vi "CallTestSuiteMethod.vi"(8 "error in":errorcluster, 10 "method":T1, 11 "TestSuite in":refnum<class "TestSuite.lvclass">) -> (0 "error out":errorcluster, 2 "Test Method Error":errorcluster, 3 "TestSuite out":refnum<class "TestSuite.lvclass">)   [LabVIEW 2011, in "TestSuite.lvclass"]
uses:
  TestSuite.lvclass
  Method--enum.ctl
  TestSuite.lvclass/TestSuite.ctl
  JKI Reuse/Filter Error Codes (Scalar)__jki_lib_error_handling -- VI Tester.vi
  Libraries/VITesterUtilities.lvlib
panel:
  # "JKI VI Tester for LabVIEW\nhttp://jkisoft.com/vi-tester\nCopyright (C) 2007-2009, JKI <info@jkisoft.com>\nALL RIGHTS RESERVED"
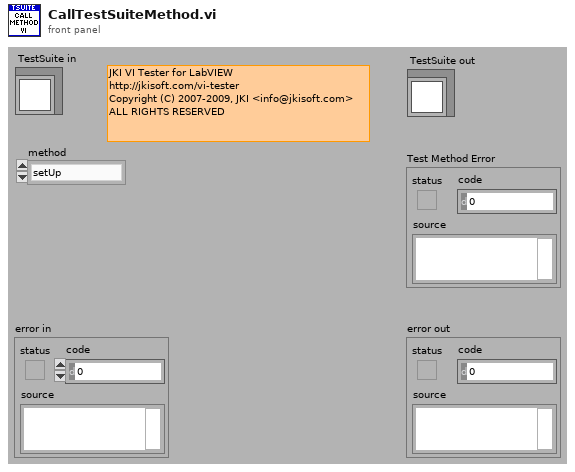
[diagram p1: front panel]
types:
  T1 = typedef "TestSuite.lvclass/Method--enum.ctl" = enum16{"setUp", "tearDown"}
  T2 = enum32{"Bad", "Idle", "Run top level", "Running"}
  T3 = cluster{"name":string, "type desc":i16[], "flat data":string}
  T4 = cluster{"name":string, "type desc":i16[], "flat data":string}[]
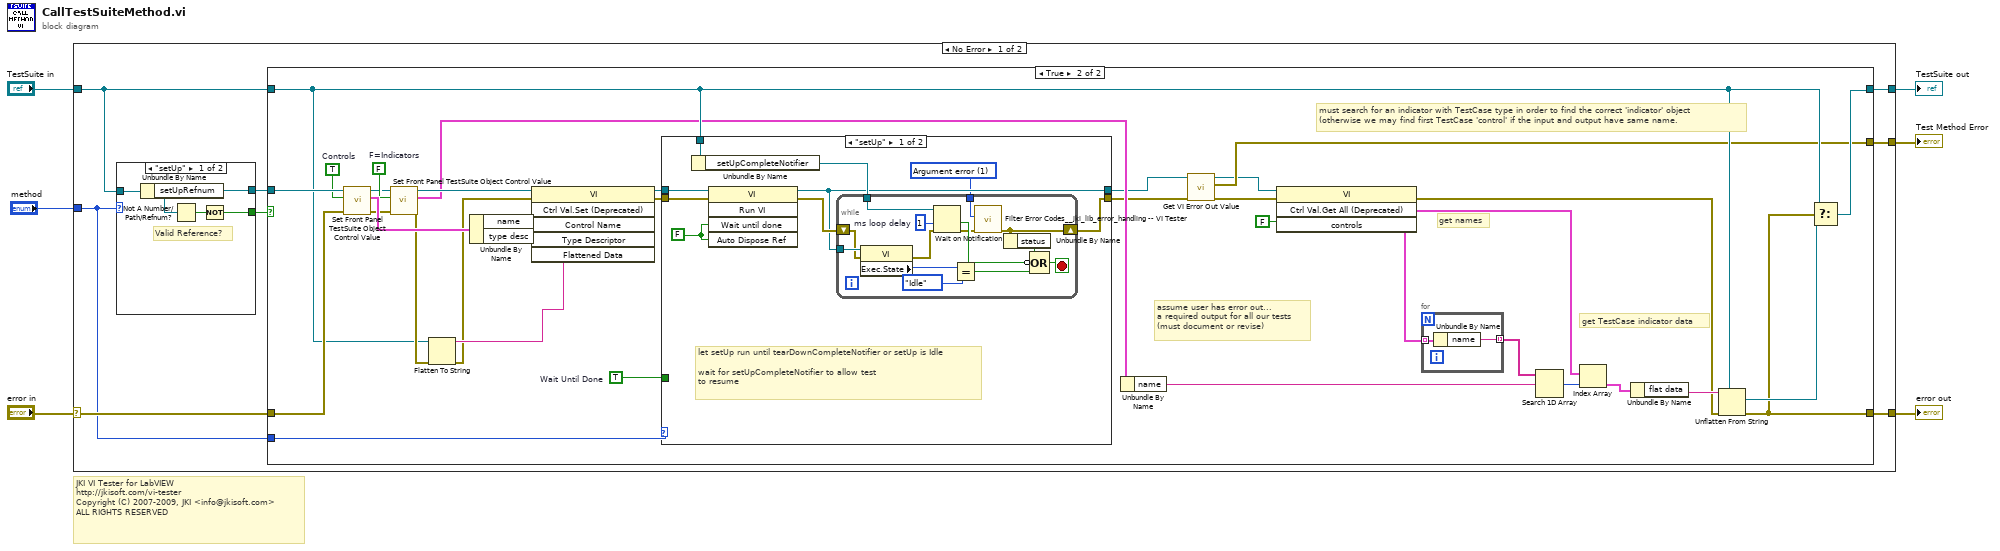
[diagram p0: block diagram]
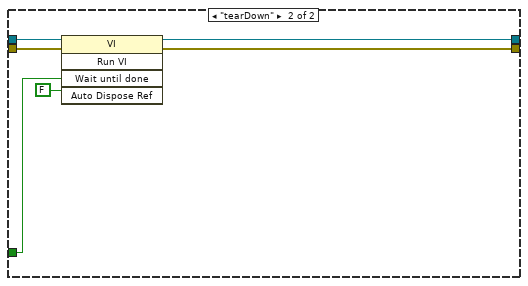
[diagram p3: hidden frame]
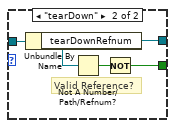
[diagram p4: hidden frame]
diagram:
  # "JKI VI Tester for LabVIEW\nhttp://jkisoft.com/vi-tester\nCopyright (C) 2007-2009, JKI <info@jkisoft.com>\nALL RIGHTS RESERVED"
  n1 = case shown="No Error" "error in" {
    selector: "error in" -> [w9 w92]
    tunnel: [w14 w91] -> w2
    tunnel: [w13 _] -> w3
    tunnel: [w12 w92] -> w4
    tunnel: "TestSuite in" -> [w11 w91]
    tunnel: "method" -> [w7 _]
    frame No Error {
      n2 = case shown="\"setUp\"" w7 {
        tunnel: w11 -> [w86 w90]
        tunnel: [w85 w89] -> w10
        tunnel: [w83 w87] -> w8
        frame "setUp" {
          # "Valid Reference?"
          n3 = Unbundle By Name(w86) -> ("setUpRefnum"=w85:refnum<vi>)
          n4 = Not A Number/Path/Refnum?(number/path/refnum=w85) -> (NaN/Path/Refnum?=w84:bool)
          n5 = Not(x=w84) -> (.not. x?=w83:bool)
        }
        frame "tearDown" {
          # "Valid Reference?"
          n6 = Unbundle By Name(w90) -> ("tearDownRefnum"=w89:refnum<vi>)
          n7 = Not A Number/Path/Refnum?(number/path/refnum=w89) -> (NaN/Path/Refnum?=w88:bool)
          n8 = Not(x=w88) -> (.not. x?=w87:bool)
        }
      }
      n9 = case shown="True" w8 {
        tunnel: [w16 w51] -> w14
        tunnel: [_ w18] -> w13
        tunnel: [w15 w26] -> w12
        tunnel: w11 -> [w16 w29]
        tunnel: w10 -> [_ w47]
        tunnel: w9 -> [w15 w38]
        tunnel: w7 -> [_ w35]
        frame False {
        }
        frame True {
          w34 = TRUE  # Wait Until Done
          w42 = FALSE  # F=Indicators
          w46 = TRUE  # Controls
          # "get TestCase indicator data"
          # "get names"
          # "must search for an indicator with TestCase type in order to find the correct 'indicator' object\n(otherwise we may find first TestCase 'control' if the input and output have same name."
          # "assume user has error out...\na required output for all our tests\n(must document or revise)"
          n10 = call "Set Front Panel TestSuite Object Control Value.vi"("error in"=w38, "Control (F: Indicator)"=w46, "vi reference"=w47) -> ("error out"=w41:errorcluster, "Control Value"=w45:T3, "dup vi reference"=w40:refnum<vi>)  [unwired: 5 in, 1 out]
          n11 = call "Set Front Panel TestSuite Object Control Value.vi"("error in"=w41, "Control (F: Indicator)"=w42, "vi reference"=w40) -> ("error out"=w37:errorcluster, "Control Value"=w25:T3, "dup vi reference"=w39:refnum<vi>)  [unwired: 5 in, 1 out]
          n12 = Flatten To String(anything=w29, error in (no error)=w37) -> (data string=w48:string, error out=w36:errorcluster)  [unwired: 2 in, 1 out]
          n13 = Unbundle By Name(w45) -> ("name"=w44:string, "type desc"=w43:i16[])
          n14 = invoke class="VI" method="Ctrl Val.Set (Deprecated)"(reference=w39, error in=w36, "Control Name"=w44, "Type Descriptor"=w43, "Flattened Data"=w48) -> (reference out=w50:refnum<vi>, error out=w49:errorcluster)  [unwired: 1 in, 4 out]
          n15 = case shown="\"setUp\"" w35 {
            tunnel: w50 -> [w62 w82]
            tunnel: w49 -> [w61 w81]
            tunnel: [w55 w80] -> w21
            tunnel: [w56 w79] -> w20
            tunnel: w34 -> [_ w77]
            tunnel: w29 -> [w59 _]
            frame "setUp" {
              w54 = 1 items=["No error", "Argument error", "Memory is full", "Out of zone", "End of file", "File already open", "Generic file I/O error", "File not found", "File permission error", "Disk is full", "Duplicate path", "Too many files open", "System feature not enabled", "Resource file not found", "Cannot add resource", "Resource not found", "Image not found", "Image memory error", "Pen does not exist", "Config type invalid", "Config token not found", "Config parse error", "Config memory error", "Bad external code format", "Bad external code offset", "External code not present", "Null window", "Destroy window error", "Null menu", "Print aborted", "Bad print record", "Print driver error", "Windows error during printing", "Memory error during printing", "Print dialog error", "Generic print error", "Invalid device refnum", "Device not found", "Device parameter error", "Device unit error", "Cannot open device", "Device call aborted", "Generic error", "Cancelled by user", "Object ID too low", "Object ID too high", "Object not in heap", "Unknown heap", "Unknown object (invalid DefProc)", "Unknown object (DefProc not in table)", "Message out of range", "Invalid (null) method", "Unknown message", "Manager call not supported", "Bad address", "Network operation in progress", "Network operation timed out", "Connection is busy", "Network attribute not supported", "Network error", "Address in use", "System out of memory", "Connection aborted", "Connection refused", "Not connected", "Already connected", "Connection closed", "Initialization error (interapplication manager)", "Bad occurrence", "Wait on unbound occurrence handler", "Occurrence queue overflow", "Datalog type conflict", "Unused", "Unrecognized type (interapplication manager)", "Memory corrupt", "Failed to make temporary DLL", "Old CIN version", "Drag socket not found", "Failed to load drop-object", "Failed to register OLE object", "Failed to release OLE object", "Format specifier type mismatch", "Unknown format specifier", "Too few format specifiers", "Too many format specifiers", "Scan failed", "Newer CIN version", "Error converting to variant", "Runtime menu error", "Password tampered", "Variant attribute not found", "Incompatible variant data type", "Event data is not available", "Event Store is not present", "Occurrence is not found", "Event Queue is not created", "Event info is not available", "Refnum passed is NULL", "Error retrieving Class GUID", "Error retrieving CoClass GUID", "Error retrieving TypeLib GUID.", "Bad built application magic bytes.", "Specific driver is different from the specific driver associated with the Logical Name.", "There is no session opened to the class driver.", "Max Error", "MAX - Error with config objects", "MAX - Error loading configuration", "MAX - Group not supported"]
              w60 = FALSE ("Auto Dispose Reference")
              # "let setUp run until tearDownCompleteNotifier or setUp is Idle\n\nwait for setUpCompleteNotifier to allow test\nto resume"
              n16 = Unbundle By Name(w59) -> ("setUpCompleteNotifier"=w58:refnum<notifier>)
              n17 = invoke class="VI" method="Run VI"(reference=w62, error in=w61, "Wait until done"=w60, "Auto Dispose Ref"=w60) -> (reference out=w55:refnum<vi>, error out=w57:errorcluster)  [unwired: 1 in, 3 out]
              n18 = while {
                tunnel: w58 -> [w76]
                tunnel: w55 -> [w74]
                shift-right: [w64] -> w56
                shift-left: w57 -> [w73]
                tunnel: w54 -> [w63]
                stop <- w66 stop-if-true
                w75 = 1  # ms loop delay
                n19 = property class="VI"(reference=w74, error in=w73) -> (error out=w72:errorcluster, "Exec.State"=w71:T2)  [unwired: 1 out]
                n20 = Wait on Notification(notifier=w76, timeout in ms (-1)=w75, error in (no error)=w72) -> (timed out?=w68:bool, error out=w65:errorcluster)  [unwired: 1 in, 2 out]
                n21 = Equal?(x=w71, y=T2."Idle") -> (x = y?=w69:bool)
                n22 = call-poly "Filter Error Codes__jki_lib_error_handling -- VI Tester.vi"("error in"=w65, "error code to filter"=w63) -> ("error out"=w64:errorcluster)  [unwired: 7 in, 2 out]
                n23 = Unbundle By Name(w64) -> ("status"=w67:bool)
                n24 = Compound Arithmetic op=OR(w67, invert w68, w69) -> (w66:bool)
              }
            }
            frame "tearDown" {
              n25 = invoke class="VI" method="Run VI"(reference=w82, error in=w81, "Wait until done"=w77, "Auto Dispose Ref"=FALSE ("Auto Dispose Reference")) -> (reference out=w80:refnum<vi>, error out=w79:errorcluster)  [unwired: 1 in, 3 out]
            }
          }
          n26 = Unbundle By Name(w25) -> ("name"=w22:string)
          n27 = call "Get VI Error Out Value.vi"("error in"=w20, "vi reference in"=w21) -> ("error out"=w19:errorcluster, "vi error out"=w18:errorcluster, "dup vi reference"=w17:refnum<vi>)  [unwired: 7 in]
          n28 = invoke class="VI" method="Ctrl Val.Get All (Deprecated)"(reference=w17, error in=w19, "controls"=FALSE ("Controls")) -> (error out=w27:errorcluster, "Get All Control Values"=w24:T4)  [unwired: 1 in, 2 out]
          n29 = for {
            tunnel: w24 -> [w53] mode=indexing
            tunnel: [w52] -> w23 mode=indexing
            n30 = Unbundle By Name(w53) -> ("name"=w52:string)
          }
          n31 = Search 1D Array(1D array=w23, element=w22) -> (index of element=w32:i32)  [unwired: 1 in]
          n32 = Index Array(array=w24, index=w32) -> (element=w31:T3)
          n33 = Unbundle By Name(w31) -> ("flat data"=w30:string)
          n34 = Unflatten From String(type=w29, binary string=w30, error in (no error)=w27) -> (value=w28:refnum<class "TestSuite.lvclass">, error out=w26:errorcluster)  [unwired: 2 in, 1 out]
          n35 = Select(t=w29, s=w26, f=w28) -> (s? t:f=w51:refnum<class "TestSuite.lvclass">)
        }
      }
    }
    frame Error {
    }
  }
  "error out" <- w4
  "Test Method Error" <- w3
  "TestSuite out" <- w2
